vi "Open.vi"(8 "error in (no error)":errorcluster, 11 "VI Reference Control in":refnum<class "VI Reference Control.lvclass">) -> (0 "error out":errorcluster, 3 "VI Reference Control out":refnum<class "VI Reference Control.lvclass">)   [LabVIEW 2016, in "VI Reference Control.lvclass"]
uses:
  VI Reference Control.lvclass
  VI Reference Control.lvclass/VI Reference Control.ctl
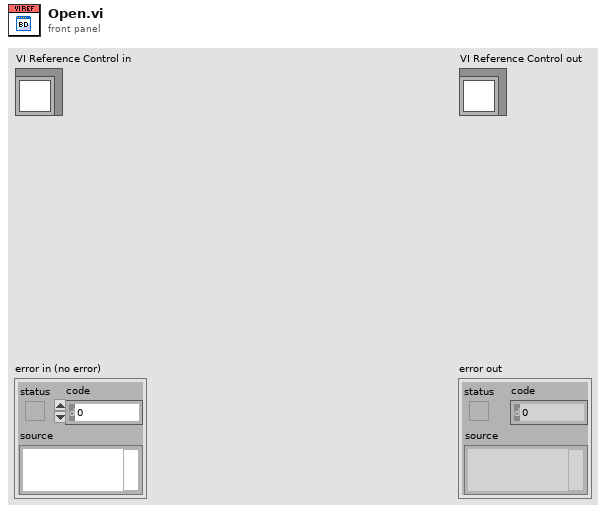
[diagram p1: front panel]
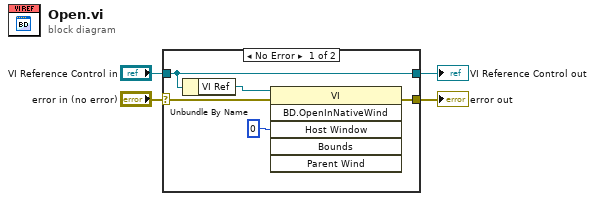
[diagram p0: block diagram]
diagram:
  n1 = case shown="No Error" "error in (no error)" {
    selector: "error in (no error)" -> [w7 w11]
    tunnel: [w6 w11] -> w3
    tunnel: [w9 w10] -> w1
    tunnel: "VI Reference Control in" -> [w9 w10]
    frame No Error {
      n2 = Unbundle By Name(w9) -> ("VI Ref"=w8:refnum<vi>)
      n3 = invoke class="VI" method="BD.OpenInNativeWind"(reference=w8, error in=w7, "Host Window"=u64 0) -> (error out=w6:errorcluster)  [unwired: 3 in, 5 out]
    }
    frame Error {
    }
  }
  "error out" <- w3
  "VI Reference Control out" <- w1
